vi "Get Todo Bookmarks.vi"(6 "open VI references? (False)":bool, 8 "error in (no error)":errorcluster, 11 "Directory to Search":path) -> (0 "error out":errorcluster, 2 "todo bookmarks":map{path, T1}(c390))   [LabVIEW 2020]
uses:
  <vilib>/Utility/miscctls.llb/LVBookmarkInfoTypeDef.ctl
panel:
  out "Errors":path[](array[path])
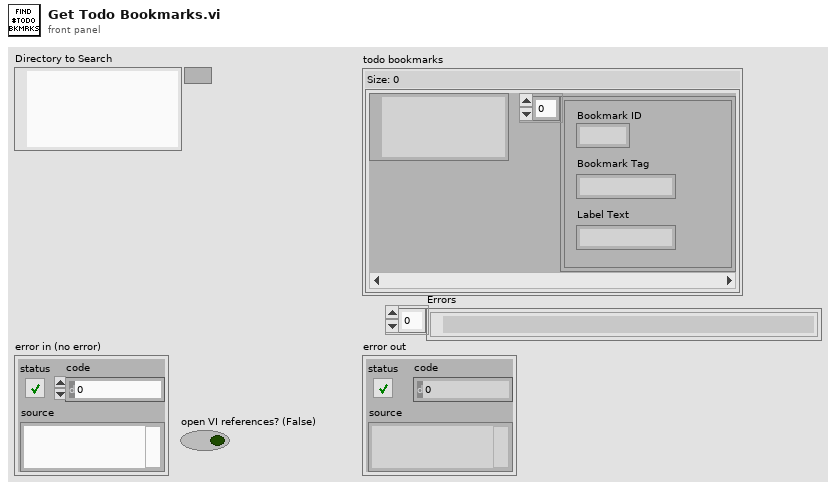
[diagram p1: front panel]
types:
  T1 = typedef "LVBookmarkInfoTypeDef.ctl" = cluster{"Bookmark ID":u32, "Bookmark Tag":string, "Label Text":string}[]
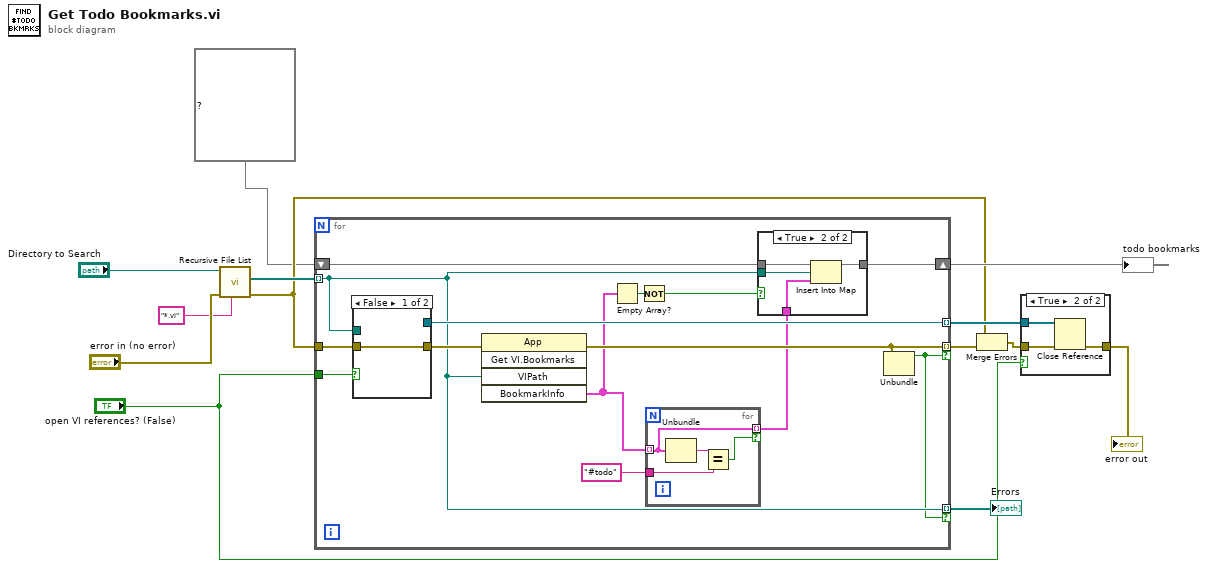
[diagram p0: block diagram]
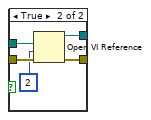
[diagram p3: hidden frame]
diagram:
  n1 = call <vilib>:"Recursive File List.vi"("pattern"="*.vi", "error in (no error)"="error in (no error)", "Folder Path"="Directory to Search") -> ("error out"=w2:errorcluster, "All Files in Dir"=w7:path[])  [unwired: 4 in, 3 out]
  n2 = for {
    tunnel: w7 -> [w15] mode=indexing
    tunnel: [w26] -> w8 mode=indexing
    shift-right: [w24] -> w13
    shift-left: map{path, T1} {} ("empty map") -> [w19]
    tunnel: w2 -> [w25]
    tunnel: [w22] -> w9 mode=indexing if=w14
    tunnel: "open VI references? (False)" -> [w16]
    tunnel: [w15] -> w3 mode=indexing if=w14
    n3 = case shown="False" w16 {
      tunnel: [w28 w33] -> w27
      tunnel: [_ w32] -> w26
      tunnel: w25 -> [w28 w31]
      tunnel: w15 -> [_ w29]
      frame False {
      }
      frame True {
        n4 = Open VI Reference(vi path=w29, options=2, error in (no error)=w31) -> (vi reference=w32:refnum<vi>, error out=w33:errorcluster)  [unwired: 3 in]
      }
    }
    n5 = invoke class="App" method="Get VI.Bookmarks"(error in=w27, "VIPath"=w15) -> (error out=w22:errorcluster, "BookmarkInfo"=w18:T1)  [unwired: 3 in, 3 out]
    n6 = Empty Array?(array=w18) -> (empty?=w23:bool)
    n7 = Not(x=w23) -> (.not. x?=w21:bool)
    n8 = for {
      tunnel: w18 -> [w35] mode=indexing
      tunnel: "#todo" ("Bookmark Tag") -> [w36]
      tunnel: [w35] -> w17 mode=indexing if=w34
      n9 = Unbundle(w35) -> ("Bookmark Tag"=w37:string)  [unwired: 2 out]
      n10 = Equal?(x=w37, y=w36) -> (x = y?=w34:bool)
    }
    n11 = case shown="True" w21 {
      tunnel: w19 -> [w38 w42]
      tunnel: [w38 w41] -> w24
      tunnel: w15 -> [_ w40]
      tunnel: w17 -> [_ w39]
      frame False {
      }
      frame True {
        n12 = Insert Into Map(map in=w42, key=w40, value=w39) -> (map out=w41:map{path, T1})  [unwired: 2 out]
      }
    }
    n13 = Unbundle(w22) -> ("status"=w14:bool)  [unwired: 2 out]
  }
  "todo bookmarks" <- w13
  "Errors" <- w3
  n14 = Merge Errors(w2, w9) -> (w11:errorcluster)
  n15 = case shown="True" "open VI references? (False)" {
    tunnel: w11 -> [w43 w46]
    tunnel: [w43 w45] -> w10
    tunnel: w8 -> [_ w44]
    frame False {
    }
    frame True {
      n16 = Close Reference(reference=w44, error in (no error)=w46) -> (error out=w45:errorcluster)
    }
  }
  "error out" <- w10
